vi "generating sequence of intructions.vi"(7 "scale maximum":u32, 8 "error in (no error)":errorcluster, 9 "átméretezett kép":i32[][](array[numeric]), 10 "új x felbontás / oszlopok száma":i32, 11 "új y felbontás / sorok száma":i32) -> (0 "error out":errorcluster, 1 "y koordináta":i32[](array[numeric]), 2 "lézer vezérlés":bool[](array[boolean]), 3 "x koordináta":i32[](array[numeric]))   [LabVIEW 2016]
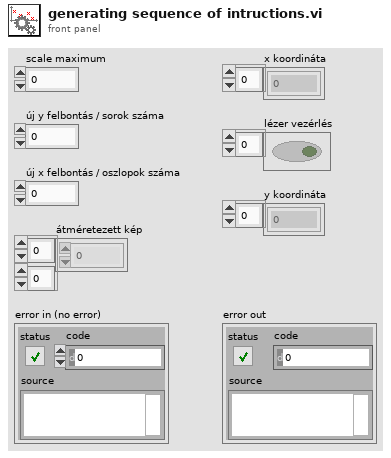
[diagram p1: front panel]
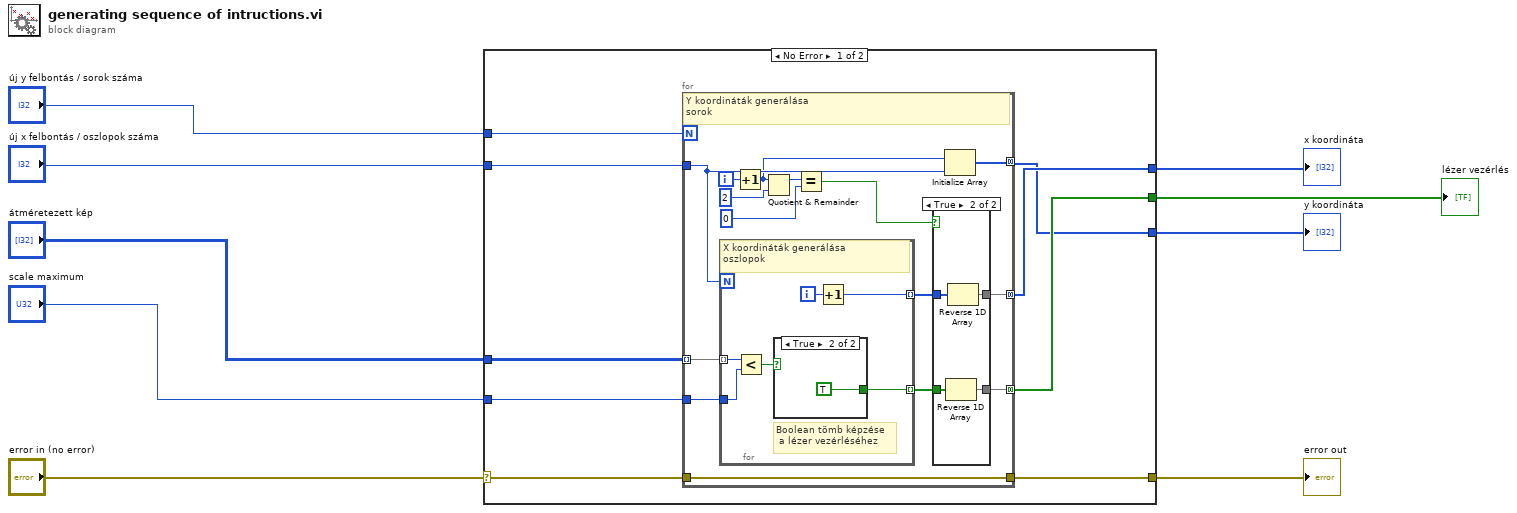
[diagram p0: block diagram]
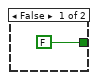
[diagram p3: hidden frame]
diagram:
  n1 = case shown="No Error" "error in (no error)" {
    selector: "error in (no error)" -> [w10 w48]
    tunnel: [w18 w48] -> w9
    tunnel: "új x felbontás / oszlopok száma" -> [w17 _]
    tunnel: "új y felbontás / sorok száma" -> [w16 _]
    tunnel: [w15 _] -> w6
    tunnel: "átméretezett kép" -> [w14 _]
    tunnel: "scale maximum" -> [w13 _]
    tunnel: [w12 _] -> w3
    tunnel: [w11 _] -> w2
    frame No Error {
      n2 = for {
        N: w16 -> [_]
        tunnel: [w29] -> w12 mode=concatenating
        tunnel: [w27] -> w11 mode=concatenating
        tunnel: [w26] -> w15 mode=concatenating
        tunnel: w17 -> [w25]
        tunnel: w14 -> [w22] mode=indexing
        tunnel: w13 -> [w21]
        tunnel: w10 -> [w19]
        tunnel: [w19] -> w18
        i -> [w28]
        # "Y koordináták generálása\nsorok"
        n3 = for {
          N: w25 -> [_]
          tunnel: [w42] -> w23 mode=indexing
          tunnel: w22 -> [w44] mode=indexing
          tunnel: w21 -> [w43]
          tunnel: [w40] -> w20 mode=indexing
          i -> [w41]
          # "Boolean tömb képzése\n a lézer vezérléséhez"
          # "X koordináták generálása\noszlopok"
          n4 = Less?(x=w44, y=w43) -> (x < y?=w45:bool)
          n5 = case shown="True" w45 {
            tunnel: [FALSE TRUE] -> w42
            frame False {
            }
            frame True {
            }
          }
          n6 = Increment(x=w41) -> (x+1=w40:i32)
        }
        n7 = Increment(x=w28) -> (x+1=w24:i32)
        n8 = Quotient & Remainder(x=w24, y=2) -> (x-y*floor(x/y)=w32:i32)  [unwired: 1 out]
        n9 = Equal?(x=w32, y=0) -> (x = y?=w30:bool)
        n10 = case shown="True" w30 {
          tunnel: w20 -> [w35 w36]
          tunnel: [w35 w39] -> w29
          tunnel: w23 -> [w34 w37]
          tunnel: [w34 w38] -> w26
          frame False {
          }
          frame True {
            n11 = Reverse 1D Array(array=w37) -> (reversed array=w38:bool[])
            n12 = Reverse 1D Array(array=w36) -> (reversed array=w39:i32[])
          }
        }
        n13 = Initialize Array(w24, w25) -> (w27:i32[])
      }
    }
    frame Error {
    }
  }
  "error out" <- w9
  "lézer vezérlés" <- w6
  "x koordináta" <- w3
  "y koordináta" <- w2
